vi "Recursive file list.vi"(8 "error in (no error)":errorcluster, 10 "Path":string, 11 "File Transfer Behavior in":refnum<class "File Transfer Behavior.lvclass">) -> (0 "error out":errorcluster, 1 "Files":string[](array[string]), 2 "Directories":string[](array[string]), 3 "File Transfer Behavior out":refnum<class "File Transfer Behavior.lvclass">)   [LabVIEW 2015, in "RT Management.lvlib" / "File Transfer Behavior.lvclass"]
doc: "Returns an array of all directories and files located within the directory at \"Path\". It does not return the directory at \"Path\" in the array of directories.\n\nIf \"Continue on error?\" is false, the VI will immediately stop at the error, returning the directories and files found up until that point. If true, the VI will ignore errors, returning all directories and files that didn't encounter an error. In both cases, if an error occurs, that error is returned."
uses:
  File Transfer Behavior.lvclass
  RT Management.lvlib
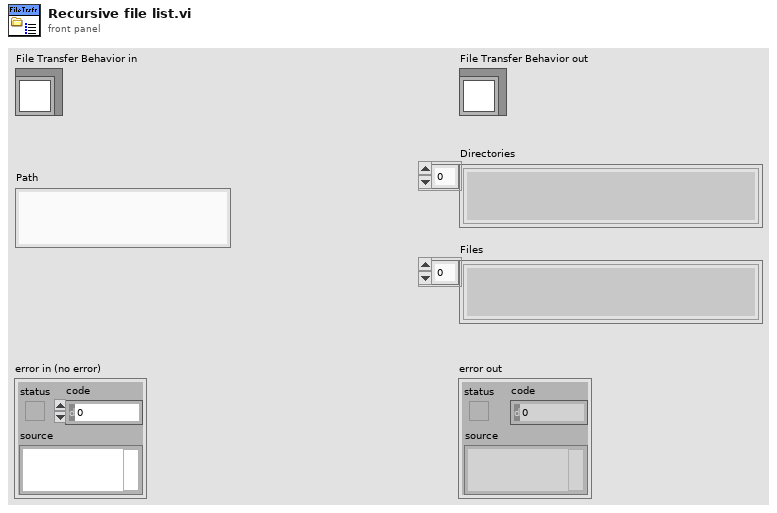
[diagram p1: front panel]
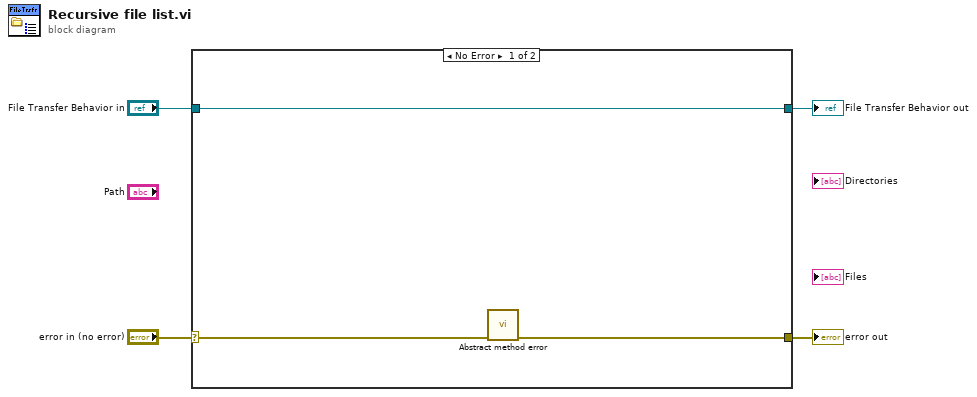
[diagram p0: block diagram]
diagram:
  n1 = case shown="No Error" "error in (no error)" {
    selector: "error in (no error)" -> [w6 w9]
    tunnel: [w5 w9] -> w3
    tunnel: [w7 w8] -> w1
    tunnel: "File Transfer Behavior in" -> [w7 w8]
    frame No Error {
      n2 = call "Abstract method error.vi"("error in (no error)"=w6) -> ("error out"=w5:errorcluster)  [unwired: 10 in]
    }
    frame Error {
    }
  }
  "error out" <- w3
  "File Transfer Behavior out" <- w1
